vi "Teleop.vi"(10 "Match Info":T1={"Autonomous Elapsed Seconds"=0.0, "TeleOp Elapsed Seconds"=0.0, "Disabled Elapsed Seconds"=0.0, "Visited Autonomous"=FALSE, "Visited TeleOp"=FALSE, "Visited Disabled"=FALSE, "Autonomous Settings"={"Autonomous Style"=enum."Independent", "VI Refnum"=refnum}}, 11 "Call Context":T2) -> ()   [LabVIEW 2017]
doc: "This VI is called for each TeleOp packet received from the DS where the robot is not disabled. It is often used to read from the joysticks and update I/O or to update setpoints for timed control loops. It should complete and return within 20 milliseconds or it may miss DS packets."
uses:
  <vilib>/Rock Robotics/WPI/DriverStation/WPI_DriverStationDerivedRobotMode.ctl
  <vilib>/Rock Robotics/WPI/DriverStation/WPI_DriverStationMatch Info.ctl
  <vilib>/Rock Robotics/WPI/Solenoid/WPI_SolenoidValue.ctl
  <vilib>/Rock Robotics/WPI/Utilities/WPI_GetSetVariantRefNum.vi
  <vilib>/Rock Robotics/Network Tables/NT Write Boolean Array.vi
  <vilib>/Rock Robotics/Network Tables/NT Write Numeric Array.vi
  <vilib>/Rock Robotics/Network Tables/NT Read Boolean.vi
  <vilib>/Rock Robotics/Network Tables/NT Read Number.vi
  <vilib>/Rock Robotics/Network Tables/NT Write Number.vi
  <vilib>/Rock Robotics/WPI/Solenoid/WPI_SolenoidSetEnum.vi
  <vilib>/Rock Robotics/WPI/Solenoid/WPI_SolenoidGetEnum.vi
panel:
  out "Boolean":bool=TRUE
  out "Numeric":dbl
  out "Sample Slider 0":dbl(slide) scale=0.0..5.0
  out "Sample Boolean 1":bool
  out "Sample Boolean 0":bool
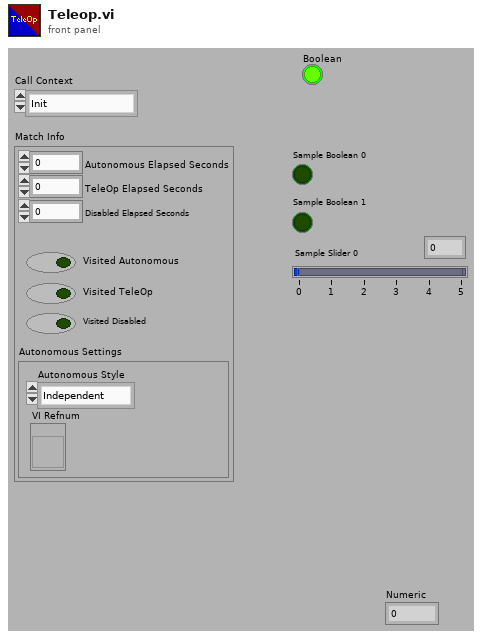
[diagram p1: front panel]
types:
  T1 = typedef "WPI_DriverStationMatch Info.ctl" = cluster{"Autonomous Elapsed Seconds":dbl, "TeleOp Elapsed Seconds":dbl, "Disabled Elapsed Seconds":dbl, "Visited Autonomous":bool, "Visited TeleOp":bool, "Visited Disabled":bool, "Autonomous Settings":cluster{"Autonomous Style":enum16{"Iterative", "Independent"}, "VI Refnum":refnum<vi>}}
  T2 = typedef "WPI_DriverStationDerivedRobotMode.ctl" = enum16{"Init", "Execute", "Stop"}
  T3 = typedef "WPI_SolenoidValue.ctl" = enum16{"Off", "On", "Forward", "Reverse"}
  T4 = typedef "WPI_RobotDriveDevRef.ctl" = cluster{"DevStatus":errorcluster, "Motors[]":T5[], "Square Inputs":bool, "Max Output":dbl}
  T5 = typedef "WPI_MotorControlDeviceRef.ctl" = cluster{"DeviceStatus":errorcluster, "Type":T6, "PWM":cluster{"PWM Channel":T7, "DeadBand":T8}, "CAN":cluster{"Device Number":u8, "SetOutput VI Ref":variant, "GetOutput VI Ref":variant, "Enable VI Ref":variant, "Disable VI Ref":variant, "Data":variant}, "Invert":bool, "DIO PWM":cluster{"PWM \"Enable\" Channel":T7, "DIOChannel":T9, "PWM Rate":dbl}}
  T6 = typedef "WPI_MotorControlType.ctl" = enum16{"PWM", "CAN", "DIO PWM"}
  T7 = typedef "FPGA_DIOPWMChannel.ctl" = enum8{"PWM 0", "PWM 1", "PWM 2", "PWM 3", "PWM 4", "PWM 5", "PWM 6", "PWM 7", "PWM 8", "PWM 9", "PWM MXP 0", "PWM MXP 1", "PWM MXP 2", "PWM MXP 3", "PWM MXP 4", "PWM MXP 5", "PWM MXP 6", "PWM MXP 7", "PWM MXP 8", "PWM MXP 9", "Invalid"}
  T8 = typedef "WPI_PWMDeadband.ctl" = cluster{"Name":string, "maxPositivePwm":i32, "minPositivePwm":i32, "centerPwm":i32, "maxNegativePwm":i32, "minNegativePwm":i32, "angularRange":u16}
  T9 = typedef "FPGA_DIOChannel.ctl" = enum8{"DIO 0", "DIO 1", "DIO 2", "DIO 3", "DIO 4", "DIO 5", "DIO 6", "DIO 7", "DIO 8", "DIO 9", "DIO MXP 0", "DIO MXP 1", "DIO MXP 2", "DIO MXP 3", "DIO MXP 4", "DIO MXP 5", "DIO MXP 6", "DIO MXP 7", "DIO MXP 8", "DIO MXP 9", "DIO MXP 10", "DIO MXP 11", "DIO MXP 12", "DIO MXP 13", "DIO MXP 14", "DIO MXP 15", "SPI Port CS1", "SPI Port CS2", "SPI Port CS3", "SPI Port MISO", "SPI Port MOSI", "Invalid"}
  T10 = typedef "WPI_JoystickDevRef.ctl" = cluster{"Device":T11}
  T11 = typedef "WPI_JoystickDeviceEnum.ctl" = enum16{"USB 0", "USB 1", "USB 2", "USB 3", "USB 4", "USB 5"}
  T12 = typedef "WPI_ServoDeviceRef.ctl" = cluster{"DeviceStatus":errorcluster, "PWM Channel":T7, "DeadBand":T8}
  T13 = cluster{"Buttons[0]":bool, "Buttons[1]":bool, "Buttons[2]":bool, "Buttons[3]":bool, "Buttons[4]":bool, "Buttons[5]":bool, "Buttons[6]":bool, "Buttons[7]":bool, "Buttons[8]":bool}
  T14 = cluster{"Axes[0]":dbl, "Axes[1]":dbl, "Axes[2]":dbl, "Axes[3]":dbl, "Axes[4]":dbl, "Axes[5]":dbl, "Axes[6]":dbl, "Axes[7]":dbl, "Axes[8]":dbl}
  T15 = typedef "WPI_GyroDevRef.ctl" = cluster{"DevStatus":errorcluster, "Analog Channel":T16, "Gain (VoltsPerDegree/Second)":dbl, "Gyro Type":enum16{"Analog", "XRS450"}, "Handle":i32, "SPI Bus":T17, "Device Found":bool, "Sample Rate":dbl, "Calibrate On Open":bool, "Offset":dbl}
  T16 = typedef "FPGA_AIChannel.ctl" = enum8{"AI 0", "AI 1", "AI 2", "AI 3", "AI MXP 0", "AI MXP 1", "AI MXP 2", "AI MXP 3", "Invalid"}
  T17 = typedef "spi_bus.ctl" = enum16{"SPI On-Board, CS0", "SPI On-Board, CS1", "SPI On-Board, CS2", "SPI On-Board, CS3", "SPI MXP", "Invalid"}
  T18 = typedef "WPI_SolenoidDevRef.ctl" = cluster{"DevStatus":errorcluster, "Pneumatics Control Module":u8, "Forward Solenoid Channel":T19, "Reverse Solenoid Channel":T19}
  T19 = typedef "WPI_SolenoidChannel.ctl" = enum8{"Solenoid 0", "Solenoid 1", "Solenoid 2", "Solenoid 3", "Solenoid 4", "Solenoid 5", "Solenoid 6", "Solenoid 7", "Invalid"}
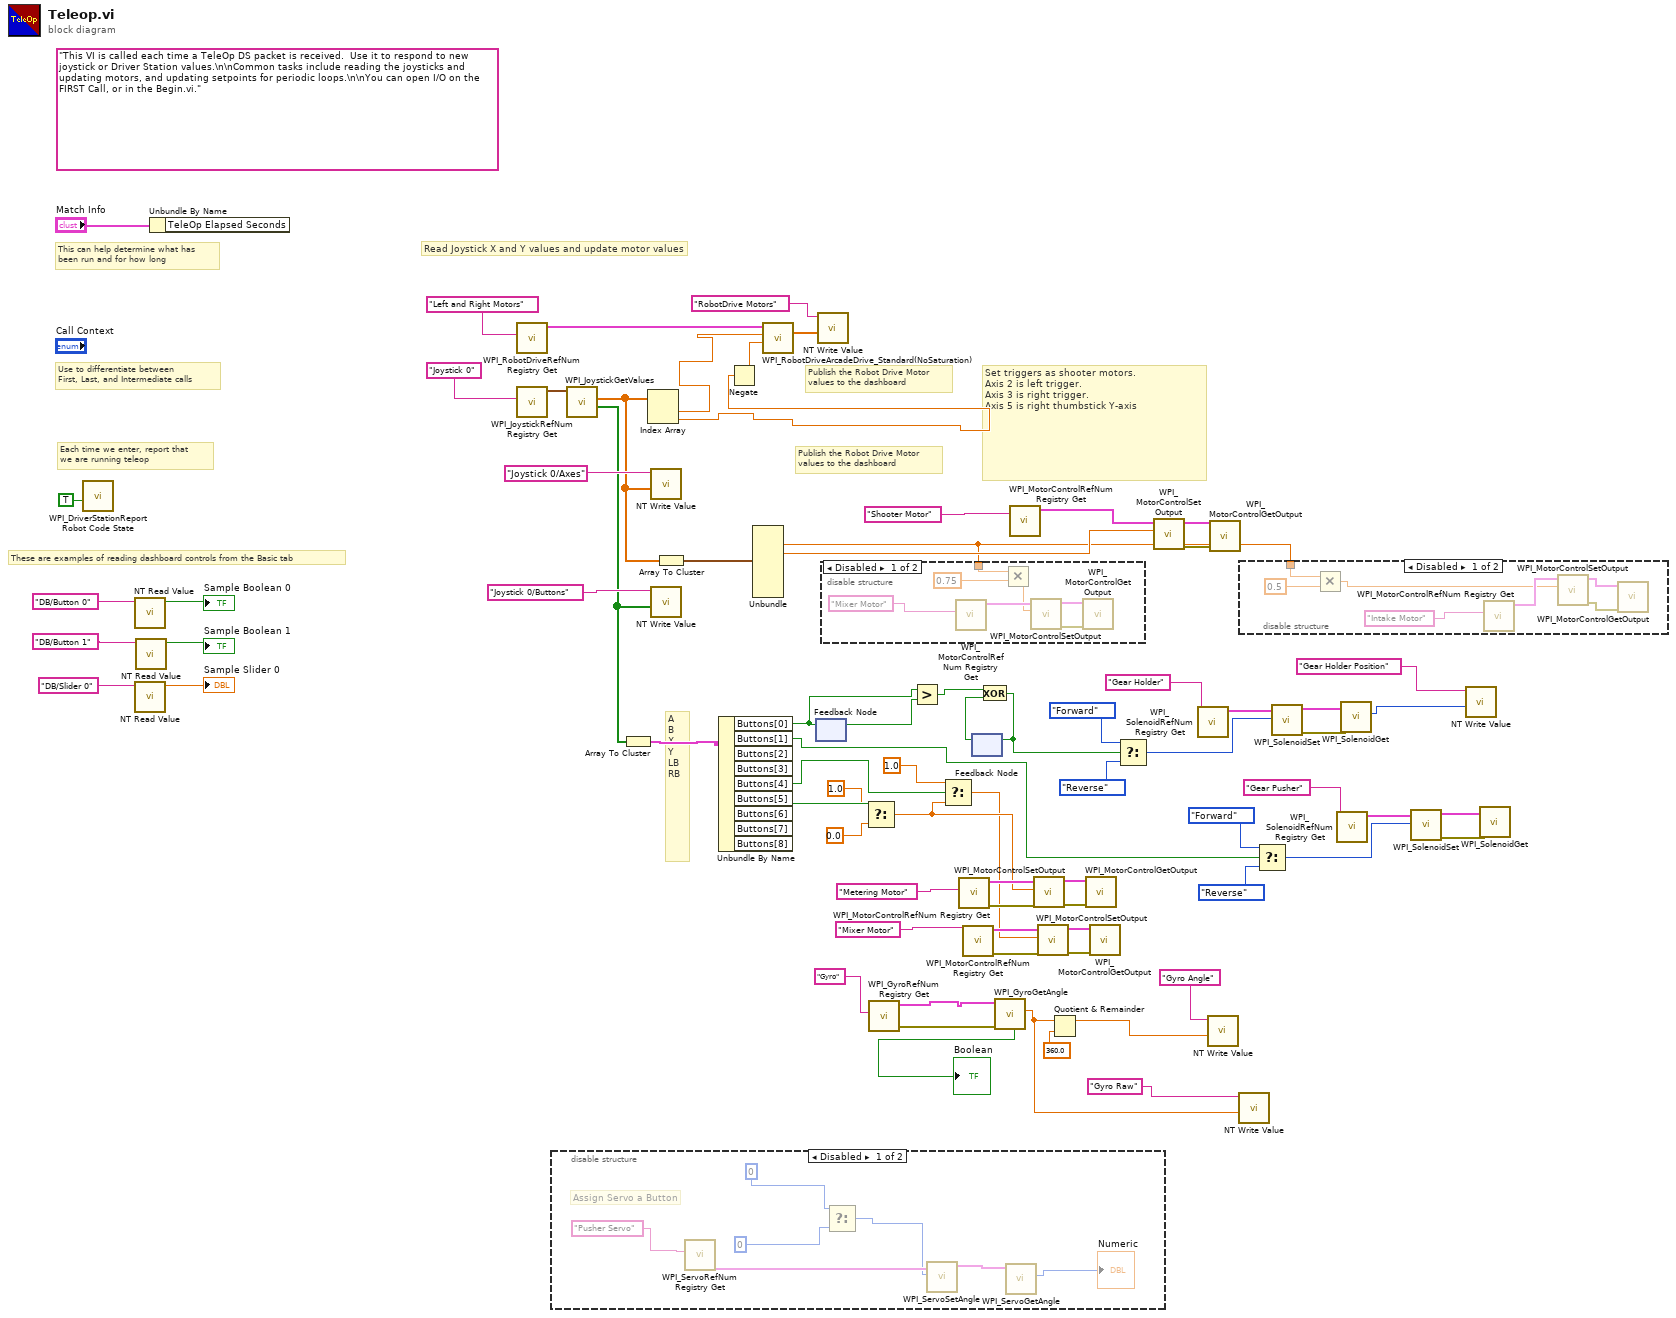
[diagram p0: block diagram]
diagram:
  (unwired) "This VI is called each time a TeleOp DS packet is received.  Use it to respond to new joystick or Driver Station values.\n\nCommon tasks include reading the joysticks and updating motors, and updating setpoints for periodic loops.\n\nYou can open I/O on the FIRST Call, or in the Begin.vi."
  # "A\nB\nX\nY\nLB\nRB"
  # "Publish the Robot Drive Motor\nvalues to the dashboard"
  # "Set triggers as shooter motors.  \nAxis 2 is left trigger.  \nAxis 3 is right trigger.\nAxis 5 is right thumbstick Y-axis"
  # "These are examples of reading dashboard controls from the Basic tab"
  # "Publish the Robot Drive Motor\nvalues to the dashboard"
  # "Each time we enter, report that\nwe are running teleop"
  # "Use to differentiate between\nFirst, Last, and Intermediate calls"
  # "This can help determine what has\nbeen run and for how long"
  # "Read Joystick X and Y values and update motor values"
  n1 = call <vilib>:"WPI_DriverStationReport Robot Code State.vi"("TeleOp"=TRUE ("Autonomous")) -> ()  [unwired: 10 in, 1 out]
  n2 = call-poly <vilib>:"NT Read Value.vi"("Name"="DB/Button 0" ("refnum name")) -> ("Boolean"=→"Sample Boolean 0":bool)  [unwired: 9 in, 1 out]
  n3 = call-poly <vilib>:"NT Read Value.vi"("Name"="DB/Slider 0" ("refnum name")) -> ("Numeric"=→"Sample Slider 0":dbl)  [unwired: 9 in, 1 out]
  n4 = call-poly <vilib>:"NT Read Value.vi"("Name"="DB/Button 1" ("refnum name")) -> ("Boolean"=→"Sample Boolean 1":bool)  [unwired: 9 in, 1 out]
  n5 = Unbundle By Name("Match Info") -> ()  [unwired: 1 out]
  n6 = call <vilib>:"WPI_RobotDriveRefNum Registry Get.vi"("refnum name"="Left and Right Motors") -> ("RobotDriveDevRef"=w75:T4)  [unwired: 1 in, 9 out]
  n7 = call <vilib>:"WPI_JoystickRefNum Registry Get.vi"("refnum name"="Joystick 0") -> ("JoystickDevRef"=w73:T10)  [unwired: 1 in, 9 out]
  n8 = disable-structure shown="Disabled" {
    frame Disabled {
      # "Assign Servo a Button"
      n9 = call <vilib>:"WPI_ServoRefNum Registry Get.vi"("refnum name"="Pusher Servo") -> ("ServoDeviceRef"=w82:T12)  [unwired: 9 in, 1 out]
      n10 = Select(t=0 ("Servo Angle, Button Pressed"), f=0 ("Servo Angle, Button Not Pressed")) -> (s? t:f=w79:i32)  [unwired: 1 in]
      n11 = call <vilib>:"WPI_ServoSetAngle.vi"("Angle"=w79, "ServoDeviceRef"=w82) -> ("ServoDeviceRef"=w84:T12)  [unwired: 1 in, 8 out]
      n12 = call <vilib>:"WPI_ServoGetAngle.vi"("ServoDeviceRef"=w84) -> ("Angle"=→"Numeric":u16)  [unwired: 1 in, 8 out]
    }
    frame Enabled {
    }
  }
  n13 = call <vilib>:"WPI_JoystickGetValues.vi"("JoystickDevRef"=w73) -> ("Buttons"=w55:bool[], "Axes"=w61:dbl[])  [unwired: 6 in, 3 out]
  n14 = Array To Cluster(array=w55) -> (cluster=w54:T13)
  n15 = Index Array(array=w61) -> (element #1=w6:dbl, element #2=w1:dbl)  [unwired: 2 in]
  n16 = call-poly <vilib>:"NT Write Value.vi"("Numeric Array"=w61, "Name"="Joystick 0/Axes") -> ()  [unwired: 9 in, 1 out]
  n17 = call-poly <vilib>:"NT Write Value.vi"("Boolean Array"=w55, "Name"="Joystick 0/Buttons") -> ()  [unwired: 9 in, 1 out]
  n18 = Array To Cluster(array=w61) -> (cluster=w60:T14)
  n19 = Unbundle By Name(w54) -> ("Buttons[0]"=w27:bool, "Buttons[1]"=w9:bool, "Buttons[4]"=w34:bool, "Buttons[5]"=w38:bool)  [unwired: 5 out]
  n20 = Negate(x=w1) -> (-x=w7:dbl)
  n21 = Unbundle(w60) -> ("Axes[2]"=w21:dbl, "Axes[3]"=w56:dbl)  [unwired: 7 out]
  n22 = call <vilib>:"WPI_RobotDriveArcadeDrive_Standard(NoSaturation).vi"("Y axis value"=w7, "X axis value"=w6, "RobotDriveDevRef"=w75) -> ("Motor Values"=w63:dbl[])  [unwired: 1 in, 7 out]
  n23 = feedback #1() -> (w30:bool)  [unwired: 1 in]
  n24 = feedback-in #1(w27) -> ()
  n25 = call-poly <vilib>:"NT Write Value.vi"("Numeric Array"=w63, "Name"="RobotDrive Motors") -> ()  [unwired: 9 in, 1 out]
  n26 = disable-structure shown="Disabled" {
    disable-tunnel: w21 -> [w87 _]
    frame Disabled {
      n27 = call <vilib>:"WPI_MotorControlRefNum Registry Get.vi"("refnum name"="Mixer Motor") -> ("MotorControlDevRef"=w90:T5)  [unwired: 9 in, 1 out]
      n28 = Multiply(x=w87, y=0.75) -> (x*y=w85:dbl)
      n29 = call <vilib>:"WPI_MotorControlSetOutput.vi"("Output"=w85, "MotorControlDevRef"=w90) -> ("error out"=w88:errorcluster, "MotorControlDevRef"=w89:T5)  [unwired: 7 in, 1 out]
      n30 = call <vilib>:"WPI_MotorControlGetOutput.vi"("error in"=w88, "MotorControlDevRef"=w89) -> ()  [unwired: 7 in, 3 out]
    }
    frame Enabled {
    }
  }
  n31 = Select(t=1.0, s=w38, f=0.0) -> (s? t:f=w32:dbl)
  n32 = call <vilib>:"WPI_GyroRefNum Registry Get.vi"("refnum name"="Gyro") -> ("error out"=w3:errorcluster, "GyroDevRef"=w2:T15)  [unwired: 9 in]
  n33 = Greater?(x=w27, y=w30) -> (0:w29:bool)
  n34 = Select(t=1.0, s=w34, f=w32) -> (s? t:f=w31:dbl)
  n35 = call <vilib>:"WPI_MotorControlRefNum Registry Get.vi"("refnum name"="Metering Motor") -> ("error out"=w48:errorcluster, "MotorControlDevRef"=w47:T5)  [unwired: 9 in]
  n36 = call <vilib>:"WPI_MotorControlRefNum Registry Get.vi"("refnum name"="Mixer Motor") -> ("error out"=w41:errorcluster, "MotorControlDevRef"=w42:T5)  [unwired: 9 in]
  n37 = feedback #2() -> (w28:bool)  [unwired: 1 in]
  n38 = Exclusive Or(1:w28, 2:w29) -> (0:w26:bool)
  n39 = feedback-in #2(w26) -> ()
  n40 = call <vilib>:"WPI_GyroGetAngle.vi"("error in"=w3, "GyroDevRef"=w2) -> ("Angle"=w4:dbl, "Calibrated?"=→"Boolean":bool)  [unwired: 5 in, 3 out]
  n41 = call <vilib>:"WPI_MotorControlRefNum Registry Get.vi"("refnum name"="Shooter Motor") -> ("MotorControlDevRef"=w58:T5)  [unwired: 9 in, 1 out]
  n42 = call <vilib>:"WPI_MotorControlSetOutput.vi"("error in (no error)"=w48, "Output"=w32, "MotorControlDevRef"=w47) -> ("error out"=w46:errorcluster, "MotorControlDevRef"=w45:T5)  [unwired: 6 in, 1 out]
  n43 = call <vilib>:"WPI_MotorControlSetOutput.vi"("error in (no error)"=w41, "Output"=w31, "MotorControlDevRef"=w42) -> ("error out"=w43:errorcluster, "MotorControlDevRef"=w44:T5)  [unwired: 6 in, 1 out]
  n44 = Quotient & Remainder(x=w4, y=360.0) -> (x-y*floor(x/y)=w17:dbl)  [unwired: 1 out]
  n45 = call <vilib>:"WPI_MotorControlGetOutput.vi"("error in"=w46, "MotorControlDevRef"=w45) -> ()  [unwired: 7 in, 3 out]
  n46 = call <vilib>:"WPI_MotorControlGetOutput.vi"("error in"=w43, "MotorControlDevRef"=w44) -> ()  [unwired: 7 in, 3 out]
  n47 = Select(t=WPI_SolenoidValue."Forward" ("Value"), s=w26, f=WPI_SolenoidValue."Reverse" ("Value")) -> (s? t:f=w49:T3)
  n48 = call <vilib>:"WPI_MotorControlSetOutput.vi"("Output"=w56, "MotorControlDevRef"=w58) -> ("error out"=w35:errorcluster, "MotorControlDevRef"=w57:T5)  [unwired: 7 in, 1 out]
  n49 = call <vilib>:"WPI_SolenoidRefNum Registry Get.vi"("refnum name"="Gear Holder") -> ("SolenoidDevRef"=w52:T18)  [unwired: 9 in, 1 out]
  n50 = call-poly <vilib>:"NT Write Value.vi"("Numeric"=w17, "Name"="Gyro Angle") -> ()  [unwired: 9 in, 1 out]
  n51 = call <vilib>:"WPI_MotorControlGetOutput.vi"("error in"=w35, "MotorControlDevRef"=w57) -> ()  [unwired: 7 in, 3 out]
  n52 = call-poly <vilib>:"NT Write Value.vi"("Numeric"=w4, "Name"="Gyro Raw") -> ()  [unwired: 9 in, 1 out]
  n53 = disable-structure shown="Disabled" {
    disable-tunnel: w21 -> [w94 _]
    frame Disabled {
      n54 = Multiply(x=w94, y=0.5) -> (x*y=w92:dbl)
      n55 = call <vilib>:"WPI_MotorControlRefNum Registry Get.vi"("refnum name"="Intake Motor") -> ("MotorControlDevRef"=w96:T5)  [unwired: 9 in, 1 out]
      n56 = call <vilib>:"WPI_MotorControlSetOutput.vi"("Output"=w92, "MotorControlDevRef"=w96) -> ("error out"=w98:errorcluster, "MotorControlDevRef"=w95:T5)  [unwired: 7 in, 1 out]
      n57 = call <vilib>:"WPI_MotorControlGetOutput.vi"("error in"=w98, "MotorControlDevRef"=w95) -> ()  [unwired: 7 in, 3 out]
    }
    frame Enabled {
    }
  }
  n58 = Select(t=WPI_SolenoidValue."Forward" ("Value"), s=w9, f=WPI_SolenoidValue."Reverse" ("Value")) -> (s? t:f=w14:T3)
  n59 = call-poly <vilib>:"WPI_SolenoidSet.vi"("Value"=w49, "SolenoidDevRef"=w52) -> ("error out"=w24:errorcluster, "SolenoidDevRef"=w25:T18)  [unwired: 8 in]
  n60 = call <vilib>:"WPI_SolenoidRefNum Registry Get.vi"("refnum name"="Gear Pusher") -> ("SolenoidDevRef"=w11:T18)  [unwired: 9 in, 1 out]
  n61 = call-poly <vilib>:"WPI_SolenoidGet.vi"("error in (no error)"=w24, "SolenoidDevRef"=w25) -> ("Value"=w23:T3)  [unwired: 7 in, 2 out]
  n62 = call-poly <vilib>:"WPI_SolenoidSet.vi"("Value"=w14, "SolenoidDevRef"=w11) -> ("error out"=w16:errorcluster, "SolenoidDevRef"=w15:T18)  [unwired: 8 in]
  n63 = call-poly <vilib>:"NT Write Value.vi"("Numeric"=w23, "Name"="Gear Holder Position") -> ()  [unwired: 9 in, 1 out]
  n64 = call-poly <vilib>:"WPI_SolenoidGet.vi"("error in (no error)"=w16, "SolenoidDevRef"=w15) -> ()  [unwired: 7 in, 3 out]
